vi "solar_voy Register (Packet).vi"(6 "Suppress Errors? (T)":bool=TRUE, 7 "Contains HDR? (F)":bool, 8 "error in (no error)":errorcluster, 9 "Override If Exists? (F)":bool, 10 "PACKET (No HDR)":T2 {"last_time" format="%<%H:%M:%S%3u %m/%d/%y>T"}, 11 "Voyager Refnum in":T1) -> (0 "error out":errorcluster, 3 "Voyager Refnum out":T1)   [LabVIEW 2018]
doc: "This registers a Voyager packet. If <b>Override If Exists?</b> is true, this overrides the existing packet. If the packet ID is 0, this generates a new ID. By default the header items are automatically added to the packet."
uses:
  solar_voy_def/solar_voy_def_ctl ITEM.ctl
  solar_voy_def/solar_voy_def_ctl PACKET.ctl
  solar_voy_def/solar_voy_def_ctl ITEM TYPE.ctl
  type/solar_type Item Type.ctl
  solar_voy_ctl Voyager Refnum.ctl
  solar_voy_def/solar_voy_def_ctl PACKET_ID.ctl
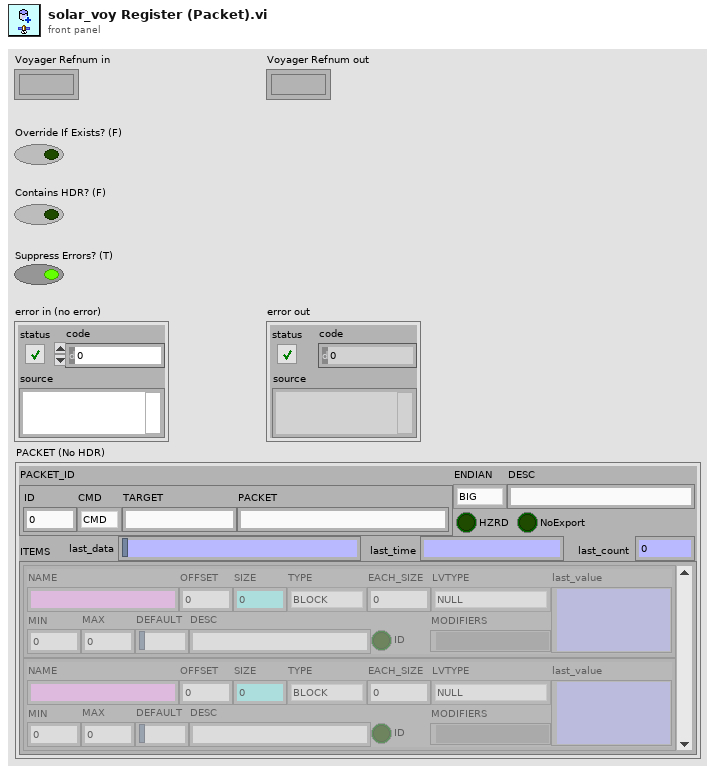
[diagram p1: front panel]
types:
  T1 = typedef "solar_voy_ctl Voyager Refnum.ctl" = refnum<k1>
  T2 = typedef "solar_voy_def_ctl PACKET.ctl" = cluster{"PACKET_ID":T3, "ENDIAN":enum8{"BIG", "LITTLE"}, "DESC":string, "HZRD":bool, "ITEMS":T4[], "NoExport":bool, "last_time":timestamp, "last_count":u32, "last_data":string}
  T3 = typedef "solar_voy_def_ctl PACKET_ID.ctl" = cluster{"ID":u16, "CMD":enum8{"CMD", "TLM"}, "TARGET":string, "PACKET":string}
  T4 = typedef "solar_voy_def_ctl ITEM.ctl" = cluster{"NAME":string, "OFFSET":i32, "SIZE":i32, "TYPE":T5, "EACH_SIZE":i32, "LVTYPE":T6, "MIN":dbl, "MAX":dbl, "DEFAULT":string, "DESC":string, "ID":bool, "MODIFIERS":variant, "last_value":variant}
  T5 = typedef "solar_voy_def_ctl ITEM TYPE.ctl" = enum8{"BLOCK", "INT", "UINT", "FLOAT", "STRING"}
  T6 = typedef "solar_type Item Type.ctl" = enum16{"NULL", "UNKNOWN", "CLUSTER", "I8", "I16", "I32", "I64", "U8", "U16", "U32", "U64", "U8_ENUM", "U16_ENUM", "U32_ENUM", "SGL", "DBL", "BOOLEAN", "STRING", "PATH", "VISA", "TAG", "TIME", "I8_1D", "I16_1D", "I32_1D", "I64_1D", "U8_1D", "U16_1D", "U32_1D", "U64_1D", "U8_ENUM_1D", "U16_ENUM_1D", "U32_ENUM_1D", "SGL_1D", "DBL_1D", "BOOLEAN_1D", "STRING_1D", "PATH_1D", "VISA_1D", "TAG_1D", "TIME_1D", "I8_2D", "I16_2D", "I32_2D", "I64_2D", "U8_2D", "U16_2D", "U32_2D", "U64_2D", "U8_ENUM_2D", "U16_ENUM_2D", "U32_ENUM_2D", "SGL_2D", "DBL_2D", "BOOLEAN_2D", "STRING_2D", "PATH_2D", "VISA_2D", "TAG_2D", "TIME_2D"}
  T7 = typedef "solar_voy_ctl Voyager.ctl" = cluster{"PACKETS":T2[], "COSMOS_Root":path, "CMD_HDR":T8, "TLM_HDR":T8, "TCPs":T9[], "VoyagerIDOffset":cluster{"VoyagerIDOffset":u16[], "Target Names":string[]}}
  T8 = typedef "solar_voy_def_ctl HDR.ctl" = cluster{"ITEMS":T4[], "LENGTH_NAME":string, "LENGTH_VALUE_OFFSET":i32, "ID_NAME":string, "ENDIAN":enum8{"BIG", "LITTLE"}, "GUID_NAME":string, "DEFAULT_TARGET":string, "DEFAULT_PACKET":string, "DEFAULT_ERROR":string}
  T9 = typedef "solar_voy_ctl TCP.ctl" = cluster{"Connected":bool, "Port":u16, "Listener":refnum<k5>, "ServerIP":string, "TCP":refnum<k5>, "Setup":T10, "VIRefnum":refnum<vi>, "TARGETS_CMD":string[], "TARGETS_TLM":string[]}
  T10 = typedef "solar_voy_ctl Port Setup.ctl" = enum8{"SERVER", "CLIENT", "SERVER_CMD", "SERVER_TLM"}
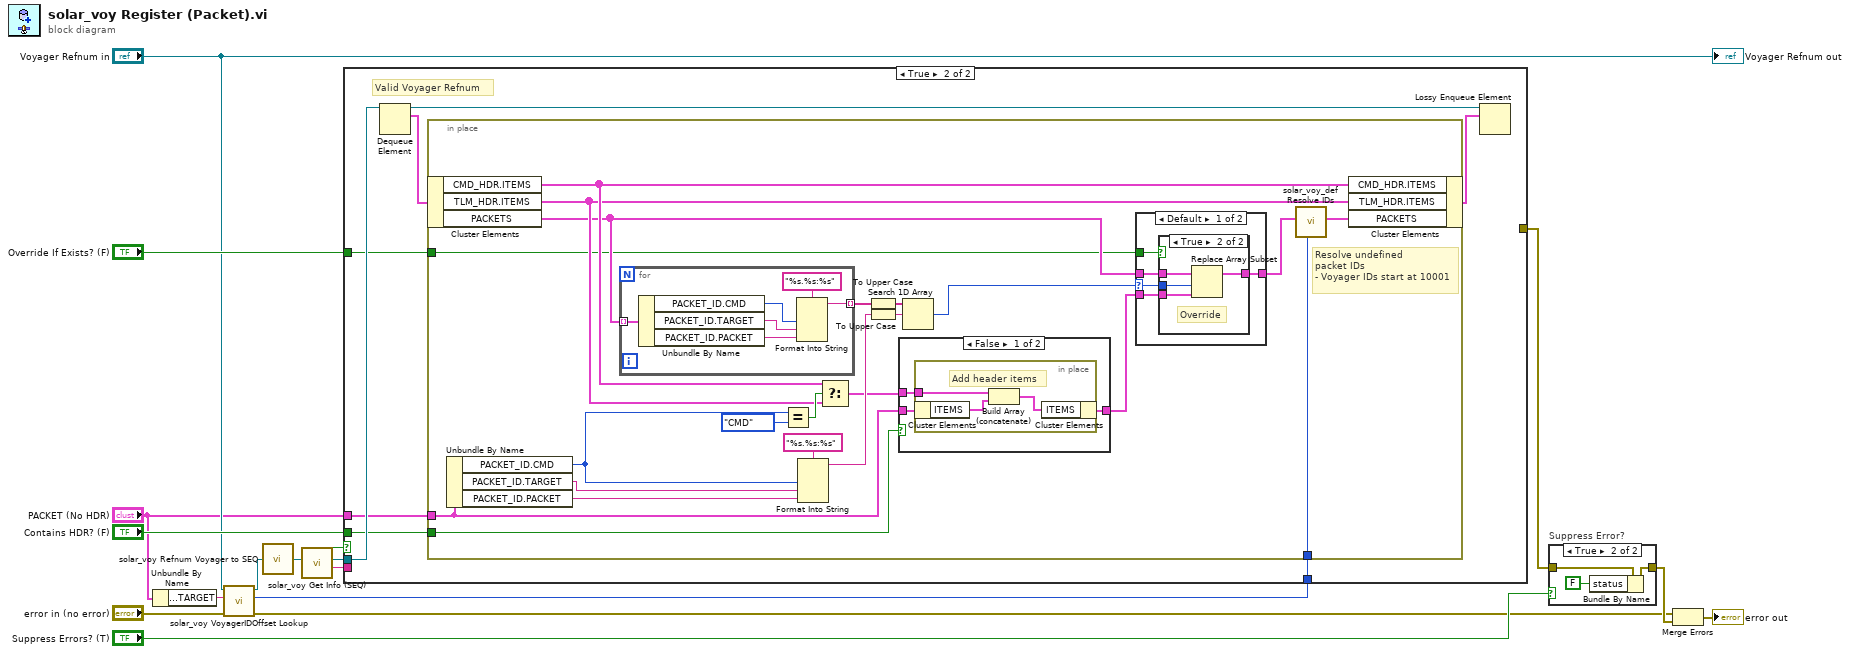
[diagram p0: block diagram]
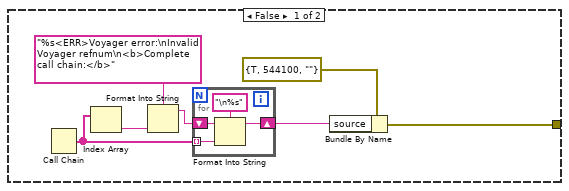
[diagram p2: hidden frame]
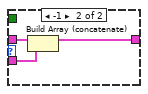
[diagram p5: hidden frame]
diagram:
  n1 = Unbundle By Name("PACKET (No HDR)") -> ("PACKET_ID.TARGET"=w1:string)
  n2 = call "solar_voy VoyagerIDOffset Lookup.vi"("error in (no error)"="error in (no error)", "Target Name"=w1, "Voyager Refnum in"="Voyager Refnum in") -> ("error out"=w6:errorcluster, "VoyagerIDOffset"=w3:u16, "Voyager Refnum out"=w4:T1)  [unwired: 6 in]
  n3 = call "solar_voy Refnum Voyager to SEQ.vi"("Voyager Refnum"=w4) -> ("Voyager SEQ"=w17:refnum<queue>)
  n4 = call "solar_voy Get Info (SEQ).vi"("Voyager SEQ in"=w17) -> ("Interface Name"=w15:string, "Voyager SEQ out"=w16:refnum<queue>, "Valid?"=w14:bool)  [unwired: 8 in]
  n5 = case shown="True" w14 {
    tunnel: w16 -> [_ w36]
    tunnel: w15 -> [_ _]
    tunnel: [w18 _] -> w12
    tunnel: "PACKET (No HDR)" -> [_ w35]
    tunnel: "Override If Exists? (F)" -> [_ w32]
    tunnel: "Contains HDR? (F)" -> [_ w31]
    tunnel: w3 -> [_ w30]
    frame False {
      n6 = Call Chain() -> (call chain=w21:string[])
      n7 = Index Array(array=w21) -> (element=w23:string)  [unwired: 1 in]
      n8 = Format Into String(format string="%s<ERR>Voyager error:\nInvalid Voyager refnum\n<b>Complete call chain:</b>", w23) -> (resulting string=w22:string)  [unwired: 2 in, 1 out]
      n9 = for {
        tunnel: w21 -> [w28] mode=indexing
        shift-right: [w27] -> w20
        shift-left: w22 -> [w26]
        n10 = Format Into String(format string="\n%s", initial string=w26, w28) -> (resulting string=w27:string)  [unwired: 1 in, 1 out]
      }
      n11 = Bundle By Name(cluster=errorcluster {"status"=TRUE, "code"=544100, "source"=""} ("error in (no error)"), "source"=w20) -> (w18:errorcluster)
    }
    frame True {
      # "Valid Voyager Refnum"
      n12 = Dequeue Element(queue=w36) -> (queue out=w29:refnum<queue>, element=w34:T7)  [unwired: 2 in, 2 out]
      n13 = in-place {
        in-place-border: w35 -> [w46]
        in-place-border: w32 -> [w41]
        in-place-border: w31 -> [w40]
        in-place-border: w30 -> [w38]
        # "Resolve undefined\npacket IDs\n- Voyager IDs start at 10001"
        n14 = in-place-cluster #1(w34) -> ("CMD_HDR.ITEMS"=w48:T4[], "TLM_HDR.ITEMS"=w47:T4[], "PACKETS"=w43:T2[])
        n15 = Unbundle By Name(w46) -> ("PACKET_ID.CMD"=w52:enum8{"CMD", "TLM"}, "PACKET_ID.TARGET"=w39:string, "PACKET_ID.PACKET"=w56:string)
        n16 = for {
          tunnel: w43 -> [w67] mode=indexing
          tunnel: [w66] -> w57 mode=indexing
          n17 = Unbundle By Name(w67) -> ("PACKET_ID.CMD"=w69:enum8{"CMD", "TLM"}, "PACKET_ID.TARGET"=w70:string, "PACKET_ID.PACKET"=w71:string)
          n18 = Format Into String(format string="%s.%s:%s", w69, w70, w71) -> (resulting string=w66:string)  [unwired: 2 in, 1 out]
        }
        n19 = Equal?(x=w52, y=enum8{"CMD", "TLM"}."CMD") -> (x = y?=w50:bool)
        n20 = Format Into String(format string="%s.%s:%s", w52, w39, w56) -> (resulting string=w54:string)  [unwired: 2 in, 1 out]
        n21 = Select(t=w48, s=w50, f=w47) -> (s? t:f=w49:T4[])
        n22 = To Upper Case(1:w57) -> (0:w44:string[])
        n23 = To Upper Case(1:w54) -> (0:w55:string)
        n24 = case shown="False" w40 {
          tunnel: w49 -> [w61 _]
          tunnel: w46 -> [w60 w65]
          tunnel: [w59 w65] -> w45
          frame False {
            n25 = in-place {
              in-place-border: w61 -> [w64]
              # "Add header items"
              n26 = in-place-cluster #2(w60) -> ("ITEMS"=w63:T4[])
              n27 = Build Array (concatenate)(w64, w63) -> (w62:T4[])
              n28 = in-place-cluster #2("ITEMS"=w62) -> (w59:T2)
            }
          }
          frame True {
            # "Already has header"
          }
        }
        n29 = Search 1D Array(1D array=w44, element=w55) -> (index of element=w58:i32)  [unwired: 1 in]
        n30 = case shown="Default" w58 {
          selector: w58 -> [w74 _]
          tunnel: [w75 w82] -> w37
          tunnel: w43 -> [w76 w84]
          tunnel: w45 -> [w73 w83]
          tunnel: w41 -> [w72 _]
          frame Default {
            n31 = case shown="True" w72 {
              tunnel: w76 -> [w77 w81]
              tunnel: [w77 w80] -> w75
              tunnel: w74 -> [_ w79]
              tunnel: w73 -> [_ w78]
              frame False {
                # "Already\nexists"
              }
              frame True {
                # "Override"
                n32 = Replace Array Subset(array=w81, new element=w78, index=w79) -> (w80:T2[])
              }
            }
          }
          frame -1 {
            n33 = Build Array (concatenate)(w84, w83) -> (w82:T2[])
          }
        }
        n34 = call "solar_voy_def Resolve IDs.vi"("VoyagerIDOffset"=w38, "PACKETS in"=w37) -> ("PACKETS out"=w42:T2[])  [unwired: 9 in]
        n35 = in-place-cluster #1("CMD_HDR.ITEMS"=w48, "TLM_HDR.ITEMS"=w47, "PACKETS"=w42) -> (w33:T7)
      }
      n36 = Lossy Enqueue Element(queue=w29, element=w33) -> ()  [unwired: 1 in, 4 out]
    }
  }
  n37 = case "Suppress Error?" shown="True" "Suppress Errors? (T)" {
    tunnel: w12 -> [w85 w88]
    tunnel: [w85 w87] -> w11
    frame False {
    }
    frame True {
      n38 = Bundle By Name(cluster=w88, "status"=FALSE) -> (w87:errorcluster)
    }
  }
  n39 = Merge Errors(w6, w11) -> (→"error out":errorcluster)
  "Voyager Refnum out" <- "Voyager Refnum in"
